vi "Write DUT Pin.vi"(8 "error in (no error)":errorcluster, 10 "DUT Pin":string, 11 "Charact Result Accessor in":refnum<class "Charact Result Accessor.lvclass">) -> (0 "error out":errorcluster, 3 "Charact Result Accessor out":refnum<class "Charact Result Accessor.lvclass">)   [LabVIEW 2023, in "RFFixtureCharact.RFPM.lvlib" / "Charact Result Accessor.lvclass"]
uses:
  Charact Result Accessor.lvclass
  Charact Result Accessor.lvclass/Charact Result Accessor.ctl
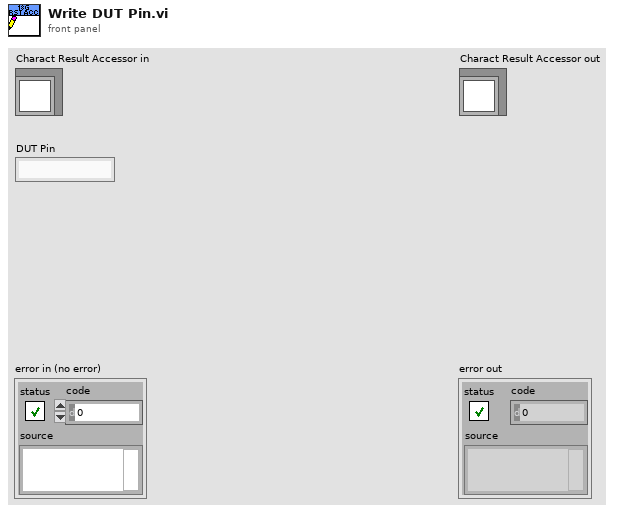
[diagram p1: front panel]
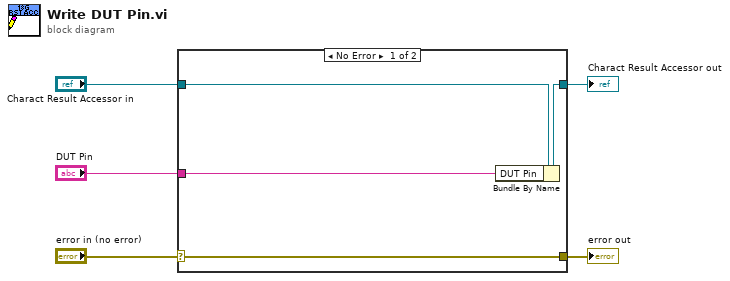
[diagram p0: block diagram]
diagram:
  n1 = case shown="No Error" "error in (no error)" {
    selector: "error in (no error)" -> [w9 w10]
    tunnel: [w9 w10] -> w4
    tunnel: [w7 w11] -> w2
    tunnel: "Charact Result Accessor in" -> [w8 w11]
    tunnel: "DUT Pin" -> [w6 _]
    frame No Error {
      n2 = Bundle By Name(cluster=w8, "DUT Pin"=w6) -> (w7:refnum<class "Charact Result Accessor.lvclass">)
    }
    frame Error {
    }
  }
  "error out" <- w4
  "Charact Result Accessor out" <- w2
